vi "Principal.vi"() -> ()   [LabVIEW 2015]
uses:
  Variable globale.vi
  <userlib>/ICNC/ICNC2.lvlib
panel:
  in  "COMMANDES MANUELLES 2 AXES":bool
  in  "Go5":bool
  in  "Go4":bool
  in  "Go3":bool
  in  "Go2":bool
  in  "Go1":bool
  in  "Vitesse 5":dbl
  in  "Vitesse 4":dbl
  in  "Vitesse 3":dbl
  in  "Vitesse 2":dbl
  in  "Vitesse 1":dbl
  in  "Angle 5":dbl
  in  "Angle 4":dbl
  in  "Angle 3":dbl
  in  "Angle 2":dbl
  in  "Angle 1":dbl
  in  "Param Systeme":bool
  out "Deverouillé":bool
  out "Connecté":bool
  out "Booléen -":bool
  out "Booléen +":bool
  out "Numérique":dbl
  in  "PARAM DLG":bool
  in  "stop moteurs":bool
  in  "Pos0":bool
  in  "stop":bool
  in  "Lancer Déplacement":bool
  in  "-":bool
  in  "+":bool
  in  "Vitesse":dbl
  in  "Angle":dbl
  in  "Vitesse Manuelle en mm/s":dbl(slide) scale=0.0..1000.0
  # "Déplacement Manuel"
  # "Exploitation"
  # "Test Déplacement"
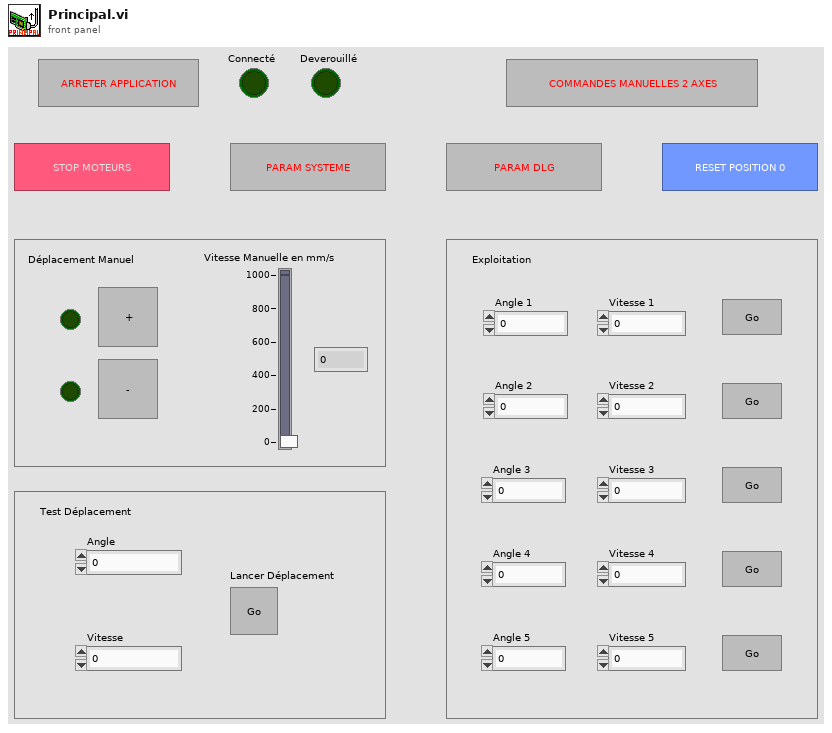
[diagram p1: front panel]
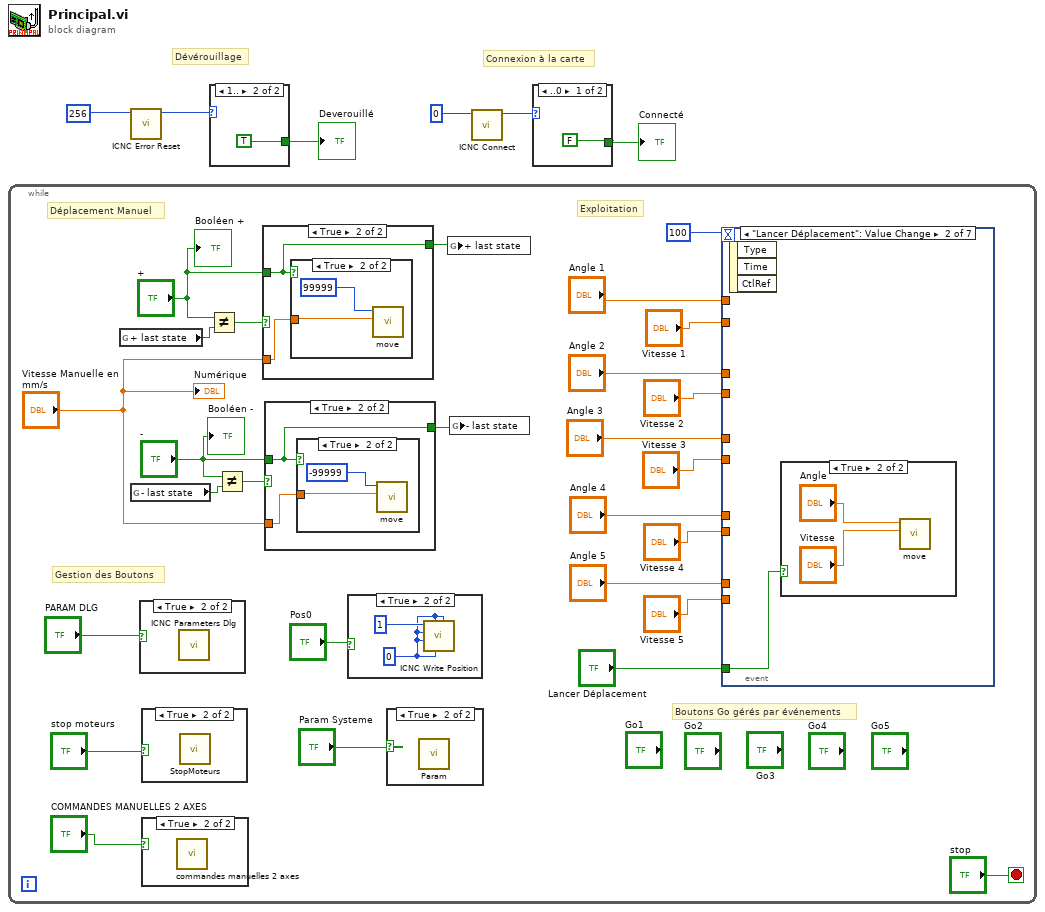
[diagram p0: block diagram]
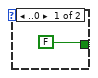
[diagram p2: hidden frame]
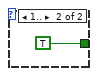
[diagram p3: hidden frame]
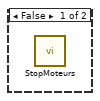
[diagram p7: hidden frame]
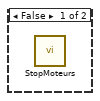
[diagram p9: hidden frame]
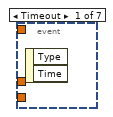
[diagram p13: hidden frame]
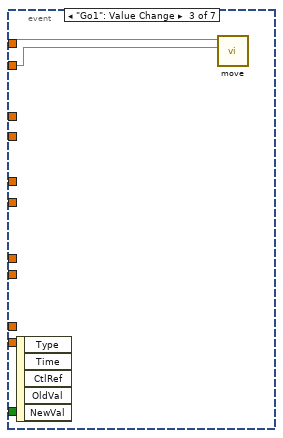
[diagram p15: hidden frame]
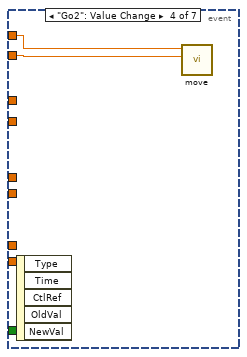
[diagram p16: hidden frame]
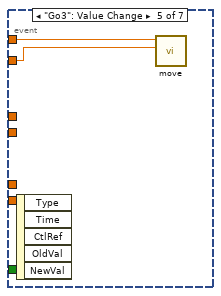
[diagram p17: hidden frame]
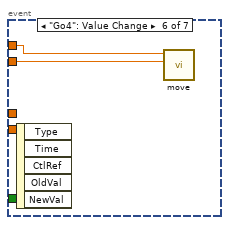
[diagram p18: hidden frame]
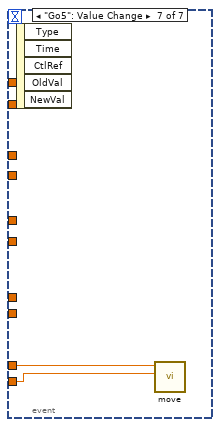
[diagram p19: hidden frame]
diagram:
  # "Connexion à la carte"
  # "Dévérouillage"
  n1 = while {
    stop <- "stop" stop-if-true
    # "Boutons Go gérés par événements"
    # "Gestion des Boutons"
    # "Déplacement Manuel"
    # "Exploitation"
    n2 = global read "Variable globale.vi" "+ last state"() -> (w15:bool)
    n3 = global read "Variable globale.vi" "- last state"() -> (w16:bool)
    n4 = case shown="True" "PARAM DLG" {
      frame False {
      }
      frame True {
        n5 = call <userlib>:"ICNC Parameters Dlg.vi"() -> ()  [unwired: 9 in, 3 out]
      }
    }
    n6 = case shown="True" "stop moteurs" {
      frame False {
      }
      frame True {
        n7 = call "StopMoteurs.vi"() -> ()  [unwired: 12 in]
      }
    }
    n8 = case shown="True" "COMMANDES MANUELLES 2 AXES" {
      frame False {
      }
      frame True {
        n9 = call "commandes manuelles 2 axes.vi"() -> ()  [unwired: 12 in]
      }
    }
    n10 = Not Equal?(x="+", y=w15) -> (x != y?=w29:bool)
    n11 = Not Equal?(x="-", y=w16) -> (x != y?=w28:bool)
    n12 = case shown="True" w29 {
      tunnel: "Vitesse Manuelle en mm/s" -> [_ w41]
      tunnel: "+" -> [w39 w40]
      tunnel: [w39 w40] -> w10
      frame False {
      }
      frame True {
        n13 = case shown="True" w40 {
          tunnel: w41 -> [_ w43]
          frame False {
            n14 = call "StopMoteurs.vi"() -> ()  [unwired: 12 in]
          }
          frame True {
            n15 = call "move.vi"("Vitesse"=w43, "Angle"=99999) -> ()  [unwired: 10 in]
          }
        }
      }
    }
    n16 = case shown="True" w28 {
      tunnel: "-" -> [w34 w35]
      tunnel: "Vitesse Manuelle en mm/s" -> [_ w36]
      tunnel: [w34 w35] -> w9
      frame False {
      }
      frame True {
        n17 = case shown="True" w35 {
          tunnel: w36 -> [_ w38]
          frame False {
            n18 = call "StopMoteurs.vi"() -> ()  [unwired: 12 in]
          }
          frame True {
            n19 = call "move.vi"("Vitesse"=w38, "Angle"=-99999) -> ()  [unwired: 10 in]
          }
        }
      }
    }
    n20 = case shown="True" "Pos0" {
      frame False {
      }
      frame True {
        w44 = 0
        n21 = call <userlib>:"ICNC Write Position.vi"("PositionB"=w44, "PositionA"=w44, "PositionZ"=w44, "PositionY"=w44, "PositionX"=w44, "Axis"=1) -> ()  [unwired: 4 in, 2 out]
      }
    }
    n22 = case shown="True" "Param Systeme" {
      frame False {
      }
      frame True {
        n23 = call "Param.vi"() -> ()  [unwired: 12 in]
      }
    }
    n24 = global write "Variable globale.vi" "+ last state"(w10) -> ()
    n25 = global write "Variable globale.vi" "- last state"(w9) -> ()
    n26 = event shown="[1] \"Lancer Déplacement\": Value Change" {
      selector: _ -> [_ _ _ _ _ _ _]
      dyn-events: _ -> [_ _ _ _ _ _ _]
      timeout: 100 -> [_ _ _ _ _ _ _]
      tunnel: "Lancer Déplacement" -> [_ w46 _ _ _ _ _]
      tunnel: "Angle 1" -> [_ _ w50 _ _ _ _]
      tunnel: "Vitesse 1" -> [_ _ w49 _ _ _ _]
      tunnel: "Angle 2" -> [_ _ _ w51 _ _ _]
      tunnel: "Vitesse 2" -> [_ _ _ w52 _ _ _]
      tunnel: "Angle 3" -> [_ _ _ _ w53 _ _]
      tunnel: "Vitesse 3" -> [_ _ _ _ w54 _ _]
      tunnel: "Angle 4" -> [_ _ _ _ _ w55 _]
      tunnel: "Vitesse 4" -> [_ _ _ _ _ w56 _]
      tunnel: "Angle 5" -> [_ _ _ _ _ _ w58]
      tunnel: "Vitesse 5" -> [_ _ _ _ _ _ w57]
      event Timeout {
        n27 = event-data() -> ()  [unwired: 1 in, 2 out]
      }
      event "Lancer Déplacement": Value Change {
        n28 = event-data() -> ()  [unwired: 1 in, 3 out]
        n29 = case shown="True" w46 {
          frame False {
          }
          frame True {
            n30 = call "move.vi"("Vitesse"="Vitesse", "Angle"="Angle") -> ()  [unwired: 10 in]
          }
        }
      }
      event "Go1": Value Change {
        n31 = event-data() -> ()  [unwired: 1 in, 5 out]
        n32 = call "move.vi"("Vitesse"=w49, "Angle"=w50) -> ()  [unwired: 10 in]
      }
      event "Go2": Value Change {
        n33 = event-data() -> ()  [unwired: 1 in, 5 out]
        n34 = call "move.vi"("Vitesse"=w52, "Angle"=w51) -> ()  [unwired: 10 in]
      }
      event "Go3": Value Change {
        n35 = event-data() -> ()  [unwired: 1 in, 5 out]
        n36 = call "move.vi"("Vitesse"=w54, "Angle"=w53) -> ()  [unwired: 10 in]
      }
      event "Go4": Value Change {
        n37 = event-data() -> ()  [unwired: 1 in, 5 out]
        n38 = call "move.vi"("Vitesse"=w56, "Angle"=w55) -> ()  [unwired: 10 in]
      }
      event "Go5": Value Change {
        n39 = event-data() -> ()  [unwired: 1 in, 5 out]
        n40 = call "move.vi"("Vitesse"=w57, "Angle"=w58) -> ()  [unwired: 10 in]
      }
    }
    "Numérique" <- "Vitesse Manuelle en mm/s"
    "Booléen -" <- "-"
    "Booléen +" <- "+"
  }
  n41 = call <userlib>:"ICNC Error Reset.vi"("ErrorBits"=256) -> ("function return"=w2:u32)  [unwired: 9 in, 1 out]
  n42 = case shown="1.." w2 {
    tunnel: [FALSE TRUE] -> w5
    frame ..0 {
    }
    frame 1.. {
    }
  }
  "Deverouillé" <- w5
  n43 = call <userlib>:"ICNC Connect.vi"("ICNC_Number"=0) -> ("function return"=w3:u32)  [unwired: 9 in, 1 out]
  n44 = case shown="..0" w3 {
    tunnel: [FALSE TRUE] -> w6
    frame ..0 {
    }
    frame 1.. {
    }
  }
  "Connecté" <- w6
